vi "ZE_Recorder_CreateVoltageOrTemp.vi"(8 "Error In":errorcluster, 9 "keep config?":bool, 10 "Array Cluster In":T1={"physical channel"="", "channel name"="", "Range"=0.0, "Terminal"=-1, "Unit"=enum."[V]", "isTemp"=FALSE, "Description"=""} {"Terminal" items=["Default"=-1, "RSE"=10083, "NRSE"=10078, "Differential"=10106, "Pseudodifferential"=12529]}, 11 "Task In":refnum<k21>) -> (0 "error out":errorcluster, 2 "Range (+/-)":dbl, 3 "Refnum out":refnum<k21>)   [LabVIEW 2025, in "ZE_Recorder.lvlib"]
doc: "ZE_Recorder_CreateVoltageOrTemp.vi\n----------------------------------------------\nThe VI creates a voltage or temp task. In case of temperature task, the parameters are set using a pop-up.\n\nInputs:\n---------------------\n- Error In : Cluster; \n- Array Cluster In : Cluster; \n- Task In : Refnum; \n\nOutputs:\n---------------------\n- error out : Cluster; \n- Range (+/-) : DBL; \n- Refnum out : Refnum; \n\n----------------------------------------------\n25.12.2017\nZühlke Engineering AG\nCH-8952 Schlieren\nwww.zuehlke.com"
uses:
  ZE_Recorder.lvlib
  ChannelCluster.ctl
  ZE_Recorder_Units.ctl
  Temperature.ctl
  ZE_Recorder_TCCluster.ctl
  ZE_Recorder_TCSource.ctl
  ZE_Recorder_TCType.ctl
  ZE_Recorder_RTDCluster.ctl
  <vilib>/DAQmx/create/channels.llb/DAQmx Create Channel (AI-Voltage-Basic).vi
  <vilib>/DAQmx/create/channels.llb/DAQmx Create Channel (AI-Temperature-Thermocouple).vi
  <vilib>/DAQmx/create/channels.llb/DAQmx Create Channel (AI-Temperature-RTD).vi
  <vilib>/DAQmx/create/channels.llb/DAQmx Create Channel (AI-Temperature-Thermistor-Vex).vi
panel:
  in  "Description":string
  # "Connector Pane"
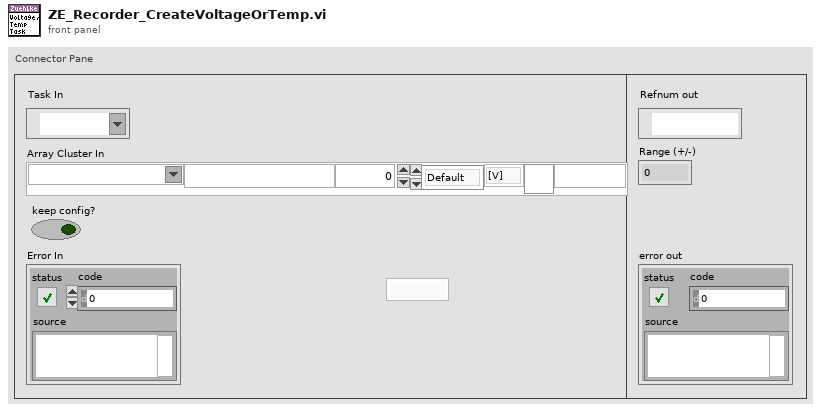
[diagram p1: front panel]
types:
  T1 = typedef "ZE_Recorder.lvlib/ChannelCluster.ctl" = cluster{"physical channel":tag, "channel name":string, "Range":dbl, "Terminal":i32, "Unit":T2, "isTemp":T3, "Description":string}
  T2 = typedef "ZE_Recorder.lvlib/ZE_Recorder_Units.ctl" = enum16{"[V]", "[A]", "[F]", "[H]", "[°C]", "[ml/s]", "[m/s]", "[bar]", "[%]", "[N]", "[?]"}
  T3 = typedef "ZE_Recorder.lvlib/Temperature.ctl" = bool
  T4 = typedef "ZE_Recorder.lvlib/ZE_Recorder_TCCluster.ctl" = cluster{"TC Cold Junction":dbl, "Cold Junction Source":T5, "TC Type":T6}
  T5 = typedef "ZE_Recorder.lvlib/ZE_Recorder_TCSource.ctl" = i32
  T6 = typedef "ZE_Recorder.lvlib/ZE_Recorder_TCType.ctl" = i32
  T7 = typedef "ZE_Recorder.lvlib/ZE_Recorder_RTDCluster.ctl" = cluster{"RTD R0":dbl, "RTD Iex":dbl, "RTD Type":i32, "RTD Config":i32}
  T8 = typedef "ZE_Recorder.lvlib/ZE_Recorder_TempParam.ctl" = cluster{"ParameterBlock":variant, "TempChannelType":T9}
  T9 = typedef "ZE_Recorder.lvlib/ZE_Recorder_TempType.ctl" = enum16{"none", "Thermocouple", "RTD", "Thermistor VE", "Thermistor CE"}
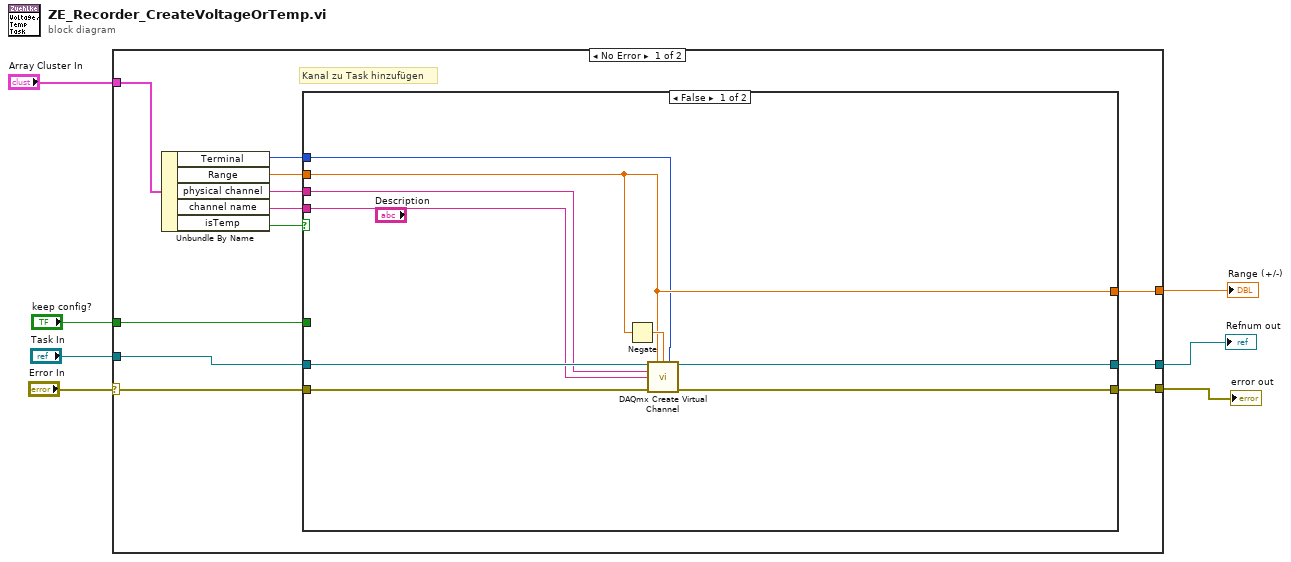
[diagram p0: block diagram]
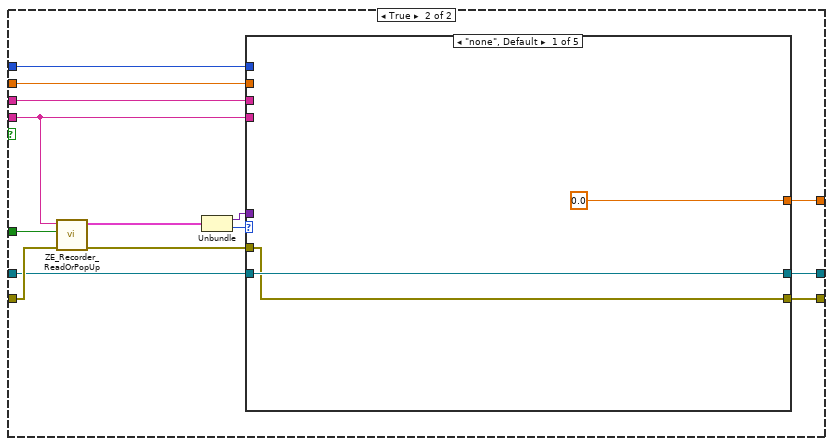
[diagram p2: hidden frame]
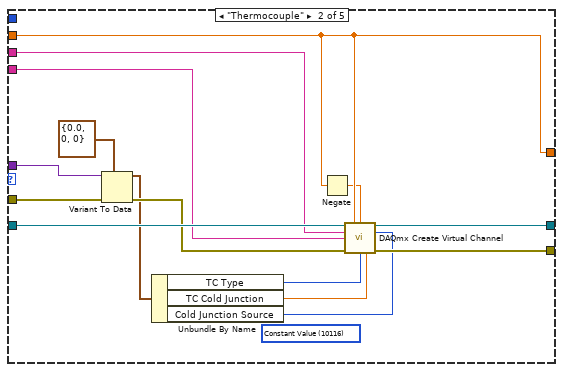
[diagram p3: hidden frame]
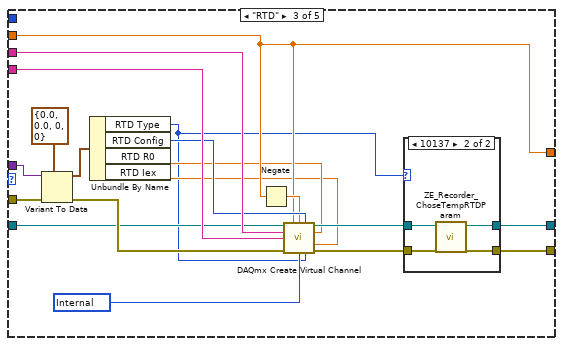
[diagram p4: hidden frame]
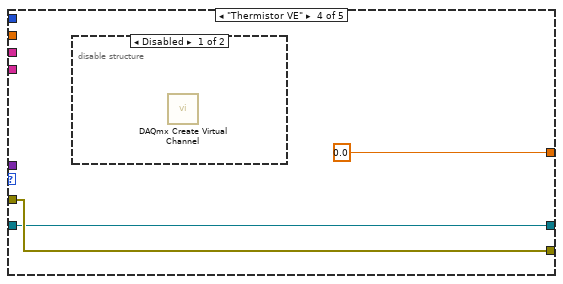
[diagram p6: hidden frame]
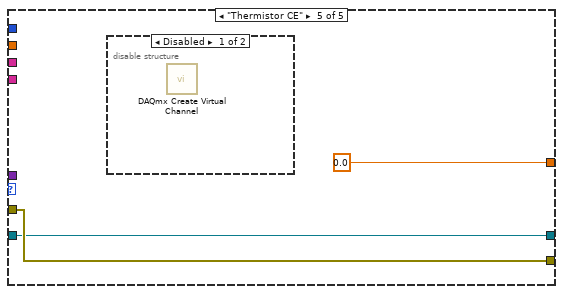
[diagram p8: hidden frame]
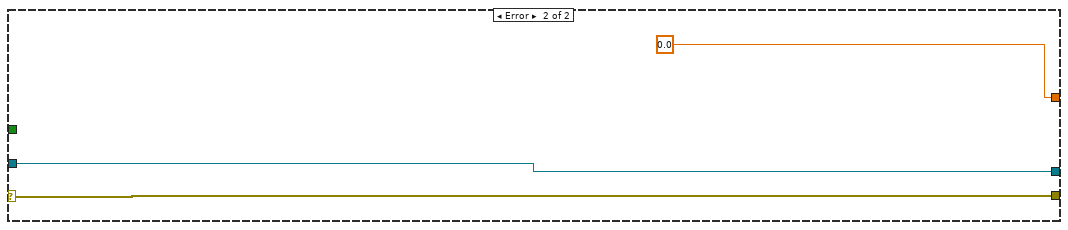
[diagram p10: hidden frame]
diagram:
  n1 = case shown="No Error" "Error In" {
    selector: "Error In" -> [w12 w94]
    tunnel: [w19 w93] -> w7
    tunnel: [w10 0.0 ("Range (+/-)")] -> w6
    tunnel: [w17 w94] -> w5
    tunnel: "Task In" -> [w16 w93]
    tunnel: "Array Cluster In" -> [w9 _]
    tunnel: "keep config?" -> [w8 _]
    frame No Error {
      # "Kanal zu Task hinzufügen"
      n2 = Unbundle By Name(w9) -> ("Terminal"=w13:i32, "Range"=w18:dbl, "physical channel"=w14:tag, "channel name"=w15:string, "isTemp"=w11:T3)
      n3 = case shown="False" w11 {
        tunnel: [w28 w31] -> w19
        tunnel: w18 -> [w21 w35]
        tunnel: [w27 w30] -> w17
        tunnel: w16 -> [w26 w37]
        tunnel: w15 -> [w25 w33]
        tunnel: w14 -> [w24 w34]
        tunnel: w13 -> [w20 w36]
        tunnel: w12 -> [w22 w42]
        tunnel: [w21 w32] -> w10
        tunnel: w8 -> [_ w29]
        frame False {
          n4 = Negate(x=w21) -> (-x=w23:dbl)
          n5 = call-poly <vilib>:"DAQmx Create Virtual Channel.vi"("task in"=w26, "maximum value"=w21, "minimum value"=w23, "input terminal configuration"=w20, "physical channels"=w24, "name to assign"=w25, "error in"=w22) -> ("task out"=w28:refnum<k21>, "error out"=w27:errorcluster)  [unwired: 7 in]
        }
        frame True {
          n6 = call "ZE_Recorder_ReadOrPopUp.vi"("error in"=w42, "Use existing"=w29, "channel name"=w33) -> ("error out"=w39:errorcluster, "channel config"=w41:T8)  [unwired: 7 in]
          n7 = Unbundle(w41) -> ("ParameterBlock"=w38:variant, "TempChannelType"=w40:T9)
          n8 = case shown="\"none\", Default" w40 {
            tunnel: w39 -> [w44 w59 w78 w88 w91]
            tunnel: w38 -> [_ w60 w79 _ _]
            tunnel: w37 -> [w45 w58 w73 w87 w90]
            tunnel: w36 -> [_ _ _ _ _]
            tunnel: w35 -> [_ w52 w70 _ _]
            tunnel: w34 -> [_ w54 w75 _ _]
            tunnel: w33 -> [_ w53 w74 _ _]
            tunnel: [0.0 ("Range (+/-)") w52 w70 0.0 ("Range (+/-)") 0.0 ("Range (+/-)")] -> w32
            tunnel: [w45 w56 w67 w87 w90] -> w31
            tunnel: [w44 w55 w65 w88 w91] -> w30
            frame "none", Default {
            }
            frame "Thermocouple" {
              (unwired) 10116 items=["Built-In"=10200, "Constant Value"=10116, "Channel"=10113] ("cjc source")
              n9 = Variant To Data(error in=w59, type=T4 {"TC Cold Junction"=0.0, "Cold Junction Source"=0, "TC Type"=0} ("output cluster"), Variant=w60) -> (data=w49:T4, error out=w57:errorcluster)
              n10 = Unbundle By Name(w49) -> ("TC Type"=w48:T6, "TC Cold Junction"=w47:dbl, "Cold Junction Source"=w46:T5)
              n11 = Negate(x=w52) -> (-x=w51:dbl)
              n12 = call-poly <vilib>:"DAQmx Create Virtual Channel.vi"("task in"=w58, "maximum value"=w52, "minimum value"=w51, "physical channels"=w54, "cjc source"=w46, "name to assign"=w53, "error in"=w57, "thermocouple type"=w48, "cjc value"=w47) -> ("task out"=w56:refnum<k21>, "error out"=w55:errorcluster)  [unwired: 5 in]
            }
            frame "RTD" {
              w69 = 10200 items=["Internal"=10200, "External"=10167, "None"=10230] ("current excitation source")
              n13 = Variant To Data(error in=w78, type=T7 {"RTD R0"=0.0, "RTD Iex"=0.0, "RTD Type"=0, "RTD Config"=0} ("output cluster"), Variant=w79) -> (data=w77:T7, error out=w76:errorcluster)
              n14 = Unbundle By Name(w77) -> ("RTD Type"=w61:i32, "RTD Config"=w72:i32, "RTD R0"=w63:dbl, "RTD Iex"=w62:dbl)
              n15 = Negate(x=w70) -> (-x=w71:dbl)
              n16 = call-poly <vilib>:"DAQmx Create Virtual Channel.vi"("task in"=w73, "maximum value"=w70, "minimum value"=w71, "resistance configuration"=w72, "physical channels"=w75, "r0"=w63, "name to assign"=w74, "current excitation value"=w62, "error in"=w76, "current excitation source"=w69, "rtd type"=w61) -> ("task out"=w68:refnum<k21>, "error out"=w66:errorcluster)  [unwired: 3 in]
              n17 = case shown="10137" w61 {
                tunnel: w68 -> [w81 w85]
                tunnel: [w81 w84] -> w67
                tunnel: w66 -> [w80 w83]
                tunnel: [w80 w82] -> w65
                frame 0, Default {
                }
                frame 10137 {
                  n18 = call "ZE_Recorder_ChoseTempRTDParam.vi"("error in (no error)"=w83, "Refnum in"=w85) -> ("error out"=w82:errorcluster, "Refnum out"=w84:refnum<k21>)  [unwired: 8 in]
                }
              }
            }
            frame "Thermistor VE" {
              n19 = disable-structure shown="Disabled" {
                frame Disabled {
                  n20 = call-poly <vilib>:"DAQmx Create Virtual Channel.vi"() -> ()  [unwired: 14 in, 2 out]
                }
                frame Enabled {
                }
              }
            }
            frame "Thermistor CE" {
              n21 = disable-structure shown="Disabled" {
                frame Disabled {
                  n22 = call-poly <vilib>:"DAQmx Create Virtual Channel.vi"() -> ()  [unwired: 14 in, 2 out]
                }
                frame Enabled {
                }
              }
            }
          }
        }
      }
    }
    frame Error {
    }
  }
  "Refnum out" <- w7
  "Range (+/-)" <- w6
  "error out" <- w5
